vi "WaveformGeneration.vi"(10 "amplitude":dbl=1.0 caption="Amplitude" format="%0.2p", 11 "signal type":T1(ring) caption="Type") -> (2 "Y":dbl[](array[numeric]), 3 "Waveform":dbl[](graph))   [LabVIEW 2014]
uses:
  <vilib>/measure/NI_MABase.lvlib
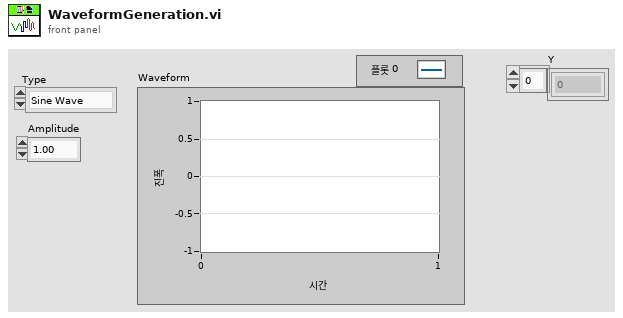
[diagram p1: front panel]
types:
  T1 = enum16{"Sine Wave", "Triangle Wave", "Square Wave", "Sawtooth Wave"}
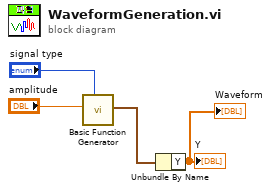
[diagram p0: block diagram]
diagram:
  n1 = call <vilib>:"Basic Function Generator.vi"("signal type"="signal type", "amplitude"="amplitude") -> ("signal out"=w2:waveform(dbl))  [unwired: 7 in, 2 out]
  n2 = Unbundle By Name(w2) -> ("Y"=→"Waveform" →"Y":dbl[])
